vi "Report Gen Item Text.vi"(8 "error in (no error)":errorcluster, 10 "Error Info":T1 {"Context"."name" items=["Method Name", "Parameter Name", "VI Name", "Control Name", "Proxy Dll Path", "Project Library Name"]; "Error Number" items=["ERR_NOERROR"=0, "ERR_ACCESS_OUTPUTFOLDER"=1, "ERR_INVALID_LIBRARYNAME"=2, "ERR_CREATE_VIWRAPPER"=3, "ERR_UNKNOWN"=201, "ERR_BAD_ARGUMENT"=202, "ERR_URL_NOTFOUND_BADWSDL"=203, "ERR_BADLYFORMATTEDURL"=204, "ERR_BADHOSTNAME"=205, "ERR_BADDIRECTORY"=206, "ERR_UNAUTHORIZEDACCESS"=207, "ERR_CREATELIBRARY"=208, "ERR_COMPILEERROR"=209]}, 11 "report":T5) -> (0 "error out":errorcluster, 2 "Text out":string, 3 "report out":T5)   [LabVIEW 2017, in "WebServiceImporter.lvlib" / "Error Handling.lvlib"]
uses:
  <vilib>/Platform/WebService/Error Handling/Error Handling.lvlib
  <resource>/importtools/NISH Report/Generate Report Object Reference.ctl
  <vilib>/Platform/WebService/Error Handling/Error/Error Info.ctl
  <vilib>/Platform/WebService/Error Handling/Error/Error Number.ctl
  <vilib>/Platform/WebService/Error Handling/Error/Context.ctl
  <vilib>/Platform/WebService/Error Handling/Error/Context Name.ctl
  <resource>/importtools/NISH Report/NISH Report.lvlib
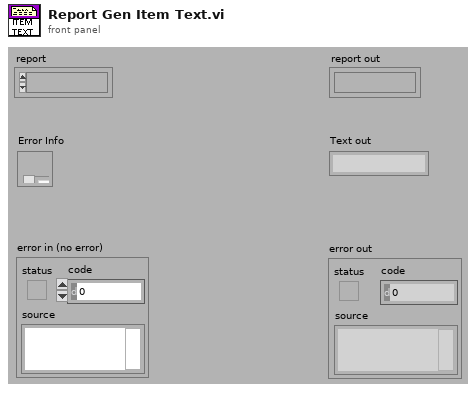
[diagram p1: front panel]
types:
  T1 = typedef "WebServiceImporter.lvlib/Error Handling.lvlib/Error Info.ctl" = cluster{"Specifics":string, "Error Number":T2, "Call Chain":string, "Context":T3}
  T2 = typedef "WebServiceImporter.lvlib/Error Handling.lvlib/Error Number.ctl" = u16
  T3 = typedef "WebServiceImporter.lvlib/Error Handling.lvlib/Context.ctl" = cluster{"name":T4, "value":string}[]
  T4 = typedef "WebServiceImporter.lvlib/Error Handling.lvlib/Context Name.ctl" = u16
  T5 = typedef "NISH Report.lvlib/Generate Report Object Reference.ctl" = refnum<k1>
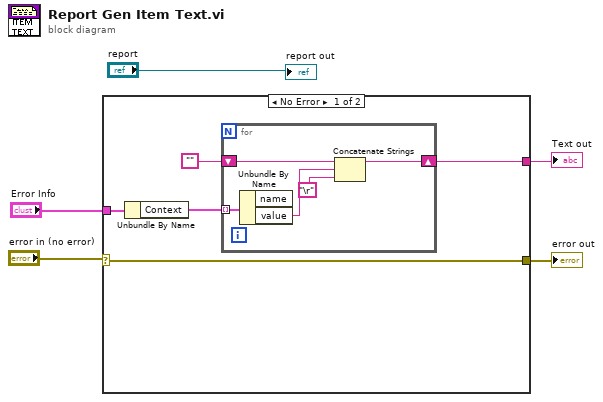
[diagram p0: block diagram]
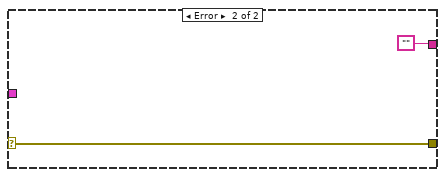
[diagram p2: hidden frame]
diagram:
  n1 = case shown="No Error" "error in (no error)" {
    selector: "error in (no error)" -> [w6 w16]
    tunnel: "Error Info" -> [w10 _]
    tunnel: [w7 ""] -> w2
    tunnel: [w6 w16] -> w1
    frame No Error {
      n2 = Unbundle By Name(w10) -> ("Context"=w9:T3)
      n3 = for {
        tunnel: w9 -> [w15] mode=indexing
        shift-right: [w11] -> w7
        shift-left: "" -> [w14]
        n4 = Unbundle By Name(w15) -> ("value"=w13:string)  [unwired: 1 out]
        n5 = Concatenate Strings(w14, w13, "\r") -> (w11:string)
      }
    }
    frame Error {
    }
  }
  "Text out" <- w2
  "error out" <- w1
  "report out" <- "report"
